vi "Lang Set Description.vi"(8 "error in (no error)":errorcluster, 10 "UI Descriptions":T1, 11 "Configuration Window in":refnum<class "Configuration Window.lvclass">) -> (0 "error out":errorcluster, 3 "Configuration Window out":refnum<class "Configuration Window.lvclass">)   [LabVIEW 2018, in "Configuration Window.lvlib" / "Configuration Window.lvclass"]
uses:
  Configuration Window.lvclass
  Framework/Framework/Const Lang Property.ctl
  Framework/Framework/Framework.lvclass
  Framework/Framework/Const Lang MainWnd Frame Title.ctl
  Framework/Framework/Const Lang MainWnd Frame Basic.ctl
  Framework/Framework/Const Lang MainWnd Frame Skill.ctl
  Framework/Framework/Const Lang MainWnd Frame bp.ctl
  Framework/Framework/Const Lang MainWnd Frame w.ctl
  Framework/Framework/Const Lang MainWnd Frame b.ctl
  Framework/Framework/Const Lang MainWnd Frame i.ctl
  Framework/Framework/Const Lang MainWnd Frame o.ctl
  Framework/Framework/Const Lang MainWnd Frame c.ctl
  Framework/Framework/Const Lang MainWnd Other.ctl
  Framework/Framework/Const Lang MainWnd Menu.ctl
  Framework/Framework/Const Lang CfgWnd Tab.ctl
  Framework/Framework/Const Lang CfgWnd Main.ctl
  Framework/Framework/Const Lang CfgWnd Path.ctl
  Framework/Framework/Const Lang CfgWnd Image.ctl
  Framework/Framework/Const Lang Setting.ctl
  Framework/Framework/Const Lang MainWnd.ctl
  Framework/Framework/Const Lang CfgWnd.ctl
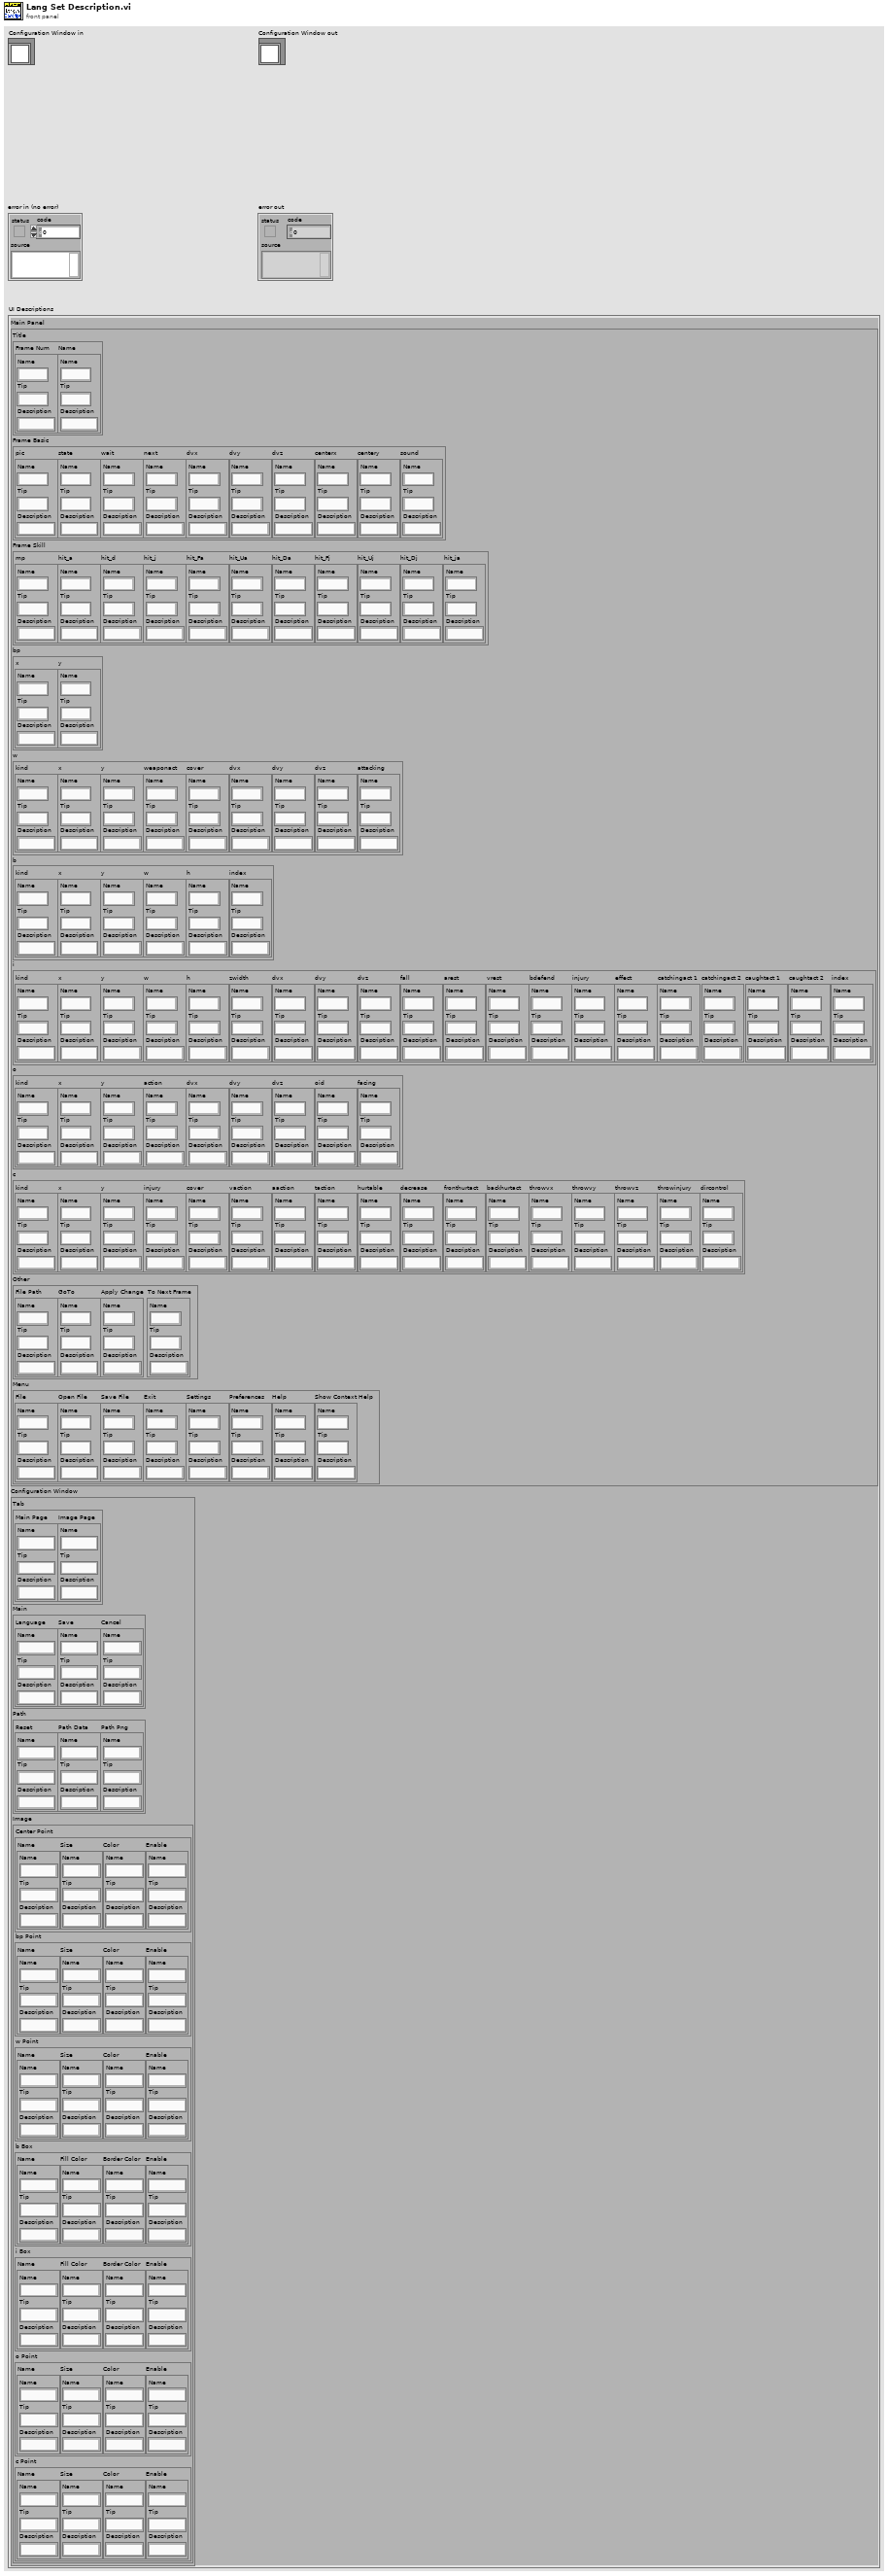
[diagram p1: front panel]
types:
  T1 = typedef "Framework.lvlib/Framework.lvclass/Const Lang Setting.ctl" = cluster{"Main Panel":T2, "Configuration Window":T15}
  T2 = typedef "Framework.lvlib/Framework.lvclass/Const Lang MainWnd.ctl" = cluster{"Title":T3, "Frame Basic":T5, "Frame Skill":T6, "bp":T7, "w":T8, "b":T9, "i":T10, "o":T11, "c":T12, "Other":T13, "Menu":T14}
  T3 = typedef "Framework.lvlib/Framework.lvclass/Const Lang MainWnd Frame Title.ctl" = cluster{"Frame Num":T4, "Name":T4}
  T4 = typedef "Framework.lvlib/Framework.lvclass/Const Lang Property.ctl" = cluster{"Name":string, "Tip":string, "Description":string}
  T5 = typedef "Framework.lvlib/Framework.lvclass/Const Lang MainWnd Frame Basic.ctl" = cluster{"pic":T4, "state":T4, "wait":T4, "next":T4, "dvx":T4, "dvy":T4, "dvz":T4, "centerx":T4, "centery":T4, "sound":T4}
  T6 = typedef "Framework.lvlib/Framework.lvclass/Const Lang MainWnd Frame Skill.ctl" = cluster{"mp":T4, "hit_a":T4, "hit_d":T4, "hit_j":T4, "hit_Fa":T4, "hit_Ua":T4, "hit_Da":T4, "hit_Fj":T4, "hit_Uj":T4, "hit_Dj":T4, "hit_ja":T4}
  T7 = typedef "Framework.lvlib/Framework.lvclass/Const Lang MainWnd Frame bp.ctl" = cluster{"x":T4, "y":T4}
  T8 = typedef "Framework.lvlib/Framework.lvclass/Const Lang MainWnd Frame w.ctl" = cluster{"kind":T4, "x":T4, "y":T4, "weaponact":T4, "cover":T4, "dvx":T4, "dvy":T4, "dvz":T4, "attacking":T4}
  T9 = typedef "Framework.lvlib/Framework.lvclass/Const Lang MainWnd Frame b.ctl" = cluster{"kind":T4, "x":T4, "y":T4, "w":T4, "h":T4, "index":T4}
  T10 = typedef "Framework.lvlib/Framework.lvclass/Const Lang MainWnd Frame i.ctl" = cluster{"kind":T4, "x":T4, "y":T4, "w":T4, "h":T4, "zwidth":T4, "dvx":T4, "dvy":T4, "dvz":T4, "fall":T4, "arest":T4, "vrest":T4, "bdefend":T4, "injury":T4, "effect":T4, "catchingact 1":T4, "catchingact 2":T4, "caughtact 1":T4, "caughtact 2":T4, "index":T4}
  T11 = typedef "Framework.lvlib/Framework.lvclass/Const Lang MainWnd Frame o.ctl" = cluster{"kind":T4, "x":T4, "y":T4, "action":T4, "dvx":T4, "dvy":T4, "dvz":T4, "oid":T4, "facing":T4}
  T12 = typedef "Framework.lvlib/Framework.lvclass/Const Lang MainWnd Frame c.ctl" = cluster{"kind":T4, "x":T4, "y":T4, "injury":T4, "cover":T4, "vaction":T4, "aaction":T4, "taction":T4, "hurtable":T4, "decrease":T4, "fronthurtact":T4, "backhurtact":T4, "throwvx":T4, "throwvy":T4, "throwvz":T4, "throwinjury":T4, "dircontrol":T4}
  T13 = typedef "Framework.lvlib/Framework.lvclass/Const Lang MainWnd Other.ctl" = cluster{"File Path":T4, "GoTo":T4, "Apply Change":T4, "To Next Frame":T4}
  T14 = typedef "Framework.lvlib/Framework.lvclass/Const Lang MainWnd Menu.ctl" = cluster{"File":T4, "Open File":T4, "Save File":T4, "Exit":T4, "Settings":T4, "Preferences":T4, "Help":T4, "Show Context Help":T4}
  T15 = typedef "Framework.lvlib/Framework.lvclass/Const Lang CfgWnd.ctl" = cluster{"Tab":T16, "Main":T17, "Path":T18, "Image":T19}
  T16 = typedef "Framework.lvlib/Framework.lvclass/Const Lang CfgWnd Tab.ctl" = cluster{"Main Page":T4, "Image Page":T4}
  T17 = typedef "Framework.lvlib/Framework.lvclass/Const Lang CfgWnd Main.ctl" = cluster{"Language":T4, "Save":T4, "Cancel":T4}
  T18 = typedef "Framework.lvlib/Framework.lvclass/Const Lang CfgWnd Path.ctl" = cluster{"Reset":T4, "Path Data":T4, "Path Png":T4}
  T19 = typedef "Framework.lvlib/Framework.lvclass/Const Lang CfgWnd Image.ctl" = cluster{"Center Point":cluster{"Name":T4, "Size":T4, "Color":T4, "Enable":T4}, "bp Point":cluster{"Name":T4, "Size":T4, "Color":T4, "Enable":T4}, "w Point":cluster{"Name":T4, "Size":T4, "Color":T4, "Enable":T4}, "b Box":cluster{"Name":T4, "Fill Color":T4, "Border Color":T4, "Enable":T4}, "i Box":cluster{"Name":T4, "Fill Color":T4, "Border Color":T4, "Enable":T4}, "o Point":cluster{"Name":T4, "Size":T4, "Color":T4, "Enable":T4}, "c Point":cluster{"Name":T4, "Size":T4, "Color":T4, "Enable":T4}}
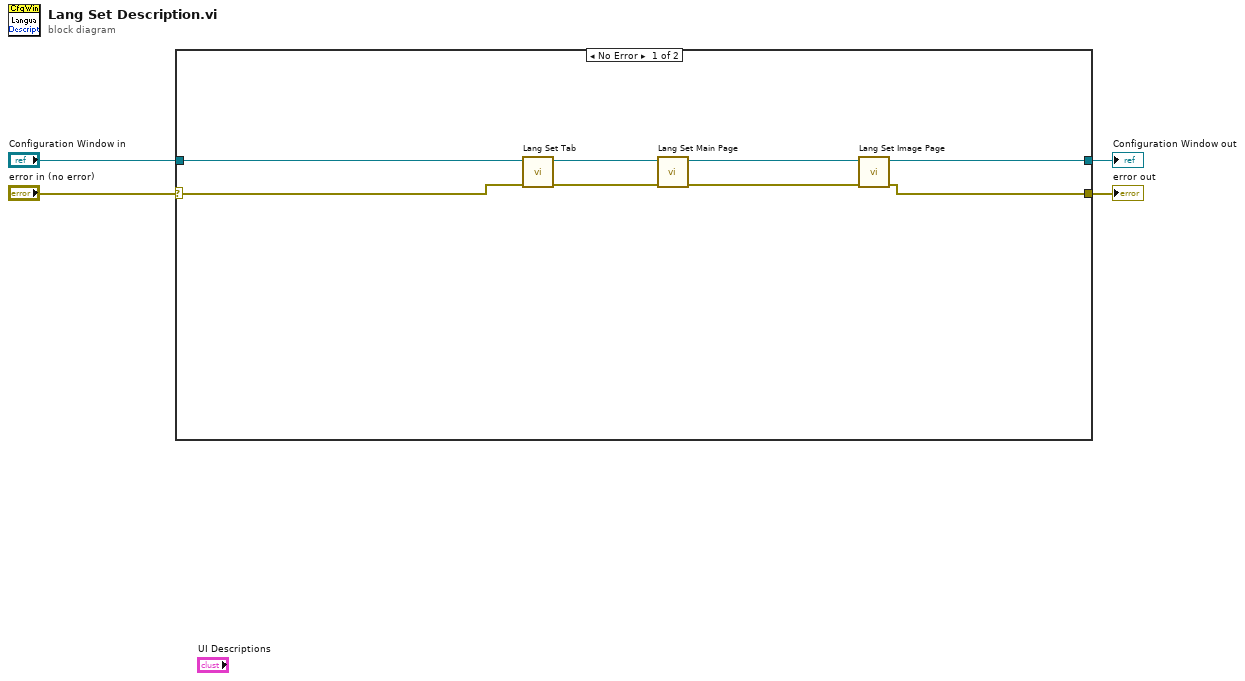
[diagram p0: block diagram]
diagram:
  n1 = case shown="No Error" "error in (no error)" {
    selector: "error in (no error)" -> [w6 w14]
    tunnel: [w5 w14] -> w3
    tunnel: [w7 w13] -> w1
    tunnel: "Configuration Window in" -> [w8 w13]
    frame No Error {
      n2 = call "Lang Set Tab.vi"("error in (no error)"=w6, "Configuration Window in"=w8) -> ("error out"=w11:errorcluster, "Configuration Window out"=w12:refnum<class "Configuration Window.lvclass">)  [unwired: 8 in]
      n3 = call "Lang Set Main Page.vi"("error in (no error)"=w11, "Configuration Window in"=w12) -> ("error out"=w9:errorcluster, "Configuration Window out"=w10:refnum<class "Configuration Window.lvclass">)  [unwired: 8 in]
      n4 = call "Lang Set Image Page.vi"("error in (no error)"=w9, "Configuration Window in"=w10) -> ("error out"=w5:errorcluster, "Configuration Window out"=w7:refnum<class "Configuration Window.lvclass">)  [unwired: 8 in]
    }
    frame Error {
    }
  }
  "error out" <- w3
  "Configuration Window out" <- w1
